vi "Master suppression revised cutoff temp.vi"() -> ()   [LabVIEW 2017]
uses:
  <vilib>/Instr/_visa.llb/VISA Configure Serial Port (Instr).vi
panel:
  in  "Ready for Testing":bool
  in  "Suppression Manual":bool
  out "Suppression Mode":bool
  out "Mode":string
  in  "Suppression Voltage":dbl
  out "Waveform Chart 2":cluster{"U":dbl}(graph)
  out "Total saving Time":dbl
  out "Waveform Chart":cluster{dbl, dbl, dbl}(graph)
  in  "Plotting Rate (ms)":u32=10 min=10 max=100 step=10
  in  "Start/Stop":bool
  out "Boolean":bool
  in  "Sampling Rate(ms)":u32=200 min=200 max=5000
  in  "Baud Rate (9600)":u32=9600
  out "Read Buffer":string
  in  "VISA resource name":refnum<visa-resource-name>
  # "DATA LOGGER with Arduino Mega"
  # "- Select VISA resource name\n- Select Baud Rate\n- Click Arrow Symbol for Start\n- Select Sampling Rate for logger\n- Click START and set name for logger \n- Click STOP to stop SAVE\n- Click Ready for Testing to start\n**Click Suppression Manual for sending \"2\" to Arduino manually"
  # "Sec"
  # "NON COMMERCIAL FOR USE"
  # "Wait for buiding .EXE"
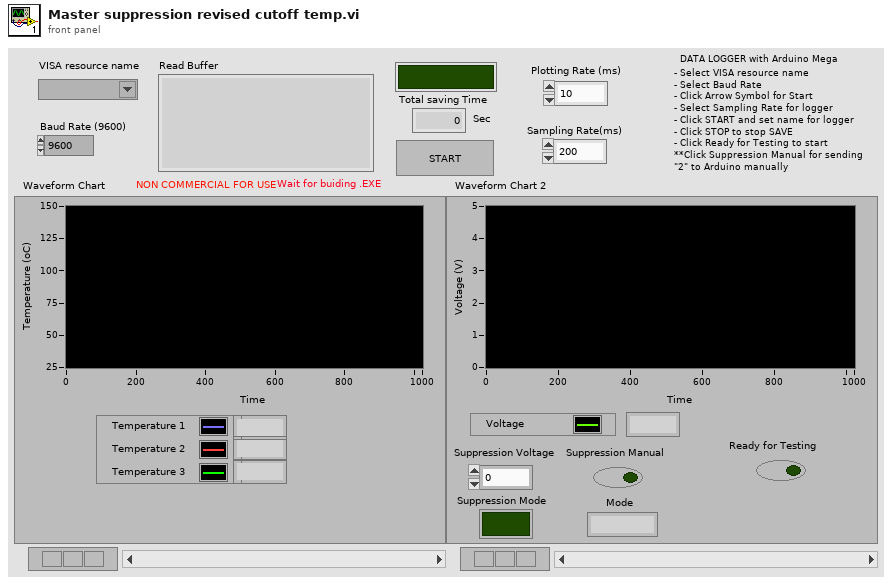
[diagram p1: front panel]
types:
  T1 = enum16{"open", "replace", "create", "open or create", "replace or create", "replace or create with confirmation"}
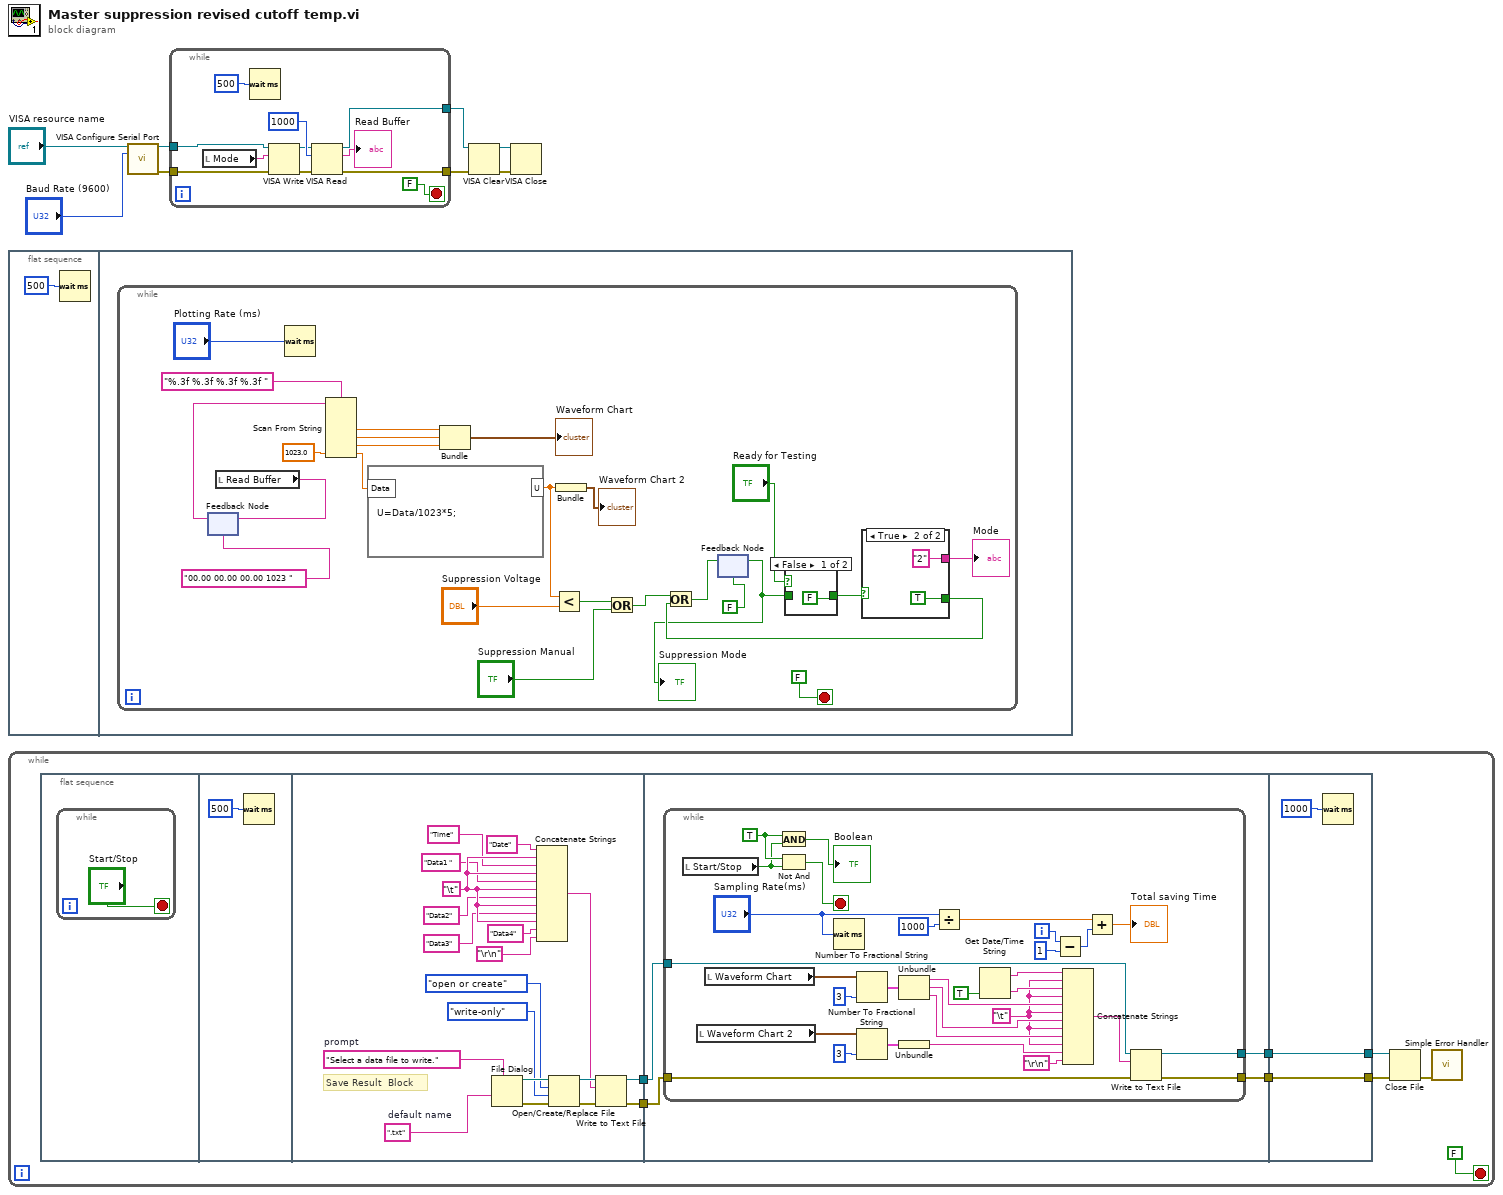
[diagram p0: block diagram]
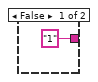
[diagram p3: hidden frame]
diagram:
  n1 = flat-sequence {
    frame #0 {
      n2 = Wait (ms)(milliseconds to wait=u32 500) -> ()  [unwired: 1 out]
    }
    frame #1 {
      n3 = while {
        stop <- FALSE ("OK Button") stop-if-true
        n4 = feedback #1("00.00 00.00 00.00 1023 " ("format string")) -> (w18:string)
        n5 = local read "Read Buffer"() -> (w19:string)
        n6 = feedback-in #1(w19) -> ()
        n7 = Wait (ms)(milliseconds to wait="Plotting Rate (ms)") -> ()  [unwired: 1 out]
        n8 = Scan From String(format string="%.3f %.3f %.3f %.3f ", input string=w18, default 4=1023.0) -> (output 1=w32:dbl, output 2=w31:dbl, output 3=w30:dbl, output 4=w26:dbl)  [unwired: 5 in, 3 out]
        n9 = formula code="U=Data/1023*5;"("Data"=w26) -> ("U"=w25:dbl)
        n10 = Bundle(w32, w31, w30) -> (→"Waveform Chart":cluster{dbl, dbl, dbl})  [unwired: 1 in]
        n11 = Less?(x=w25, y="Suppression Voltage") -> (x < y?=w21:bool)
        n12 = Bundle("U"=w25) -> (→"Waveform Chart 2":cluster{"U":dbl})  [unwired: 1 in]
        n13 = Or(x=w21, y="Suppression Manual") -> (x .or. y?=w16:bool)
        n14 = feedback #2(FALSE) -> (w12:bool)
        "Suppression Mode" <- w12
        n15 = case shown="False" "Ready for Testing" {
          tunnel: w12 -> [_ w36]
          tunnel: [FALSE w36] -> w11
          frame False {
          }
          frame True {
          }
        }
        n16 = case shown="True" w11 {
          tunnel: ["1" "2"] -> w23
          tunnel: [_ TRUE] -> w15
          frame False {
          }
          frame True {
          }
        }
        "Mode" <- w23
        n17 = Or(x=w16, y=w15) -> (x .or. y?=w14:bool)
        n18 = feedback-in #2(w14) -> ()
      }
    }
  }
  n19 = while {
    stop <- FALSE ("OK Button") stop-if-true
    n20 = flat-sequence {
      tunnel: [w52] -> w47
      tunnel: [w51] -> w46
      tunnel: w47 -> [w72]
      tunnel: w46 -> [w71]
      tunnel: [w70] -> w45
      tunnel: [w69] -> w44
      tunnel: [w106] -> w42
      tunnel: w45 -> [w106]
      tunnel: w44 -> [w105]
      tunnel: [w105] -> w41
      frame #0 {
        n21 = while {
          stop <- "Start/Stop" stop-if-true
        }
      }
      frame #1 {
        n22 = Wait (ms)(milliseconds to wait=u32 500) -> ()  [unwired: 1 out]
      }
      frame #2 {
        w60 = ".txt"  # default name
        w61 = "Select a data file to write."  # prompt
        w58 = "\t"
        # "Save Result  Block"
        n23 = File Dialog(7:w61, 9:w60) -> (0:w66:errorcluster, 3:w65:path)  [unwired: 5 in, 2 out]
        n24 = Concatenate Strings("Date", w58, "Time", w58, "Data1 ", w58, "Data2", w58, "Data3", w58, "Data4", "\r\n") -> (w64:string)
        n25 = Open/Create/Replace File(file path (use dialog)=w65, error in=w66, operation (0:open)=T1."open or create", access (0:read/write)=enum16{"read/write", "read-only", "write-only"}."write-only") -> (refnum out=w68:refnum<file>, error out=w67:errorcluster)  [unwired: 2 in, 1 out]
        n26 = Write to Text File(file (use dialog)=w68, text=w64, error in=w67) -> (refnum out=w52:refnum<file>, error out=w51:errorcluster)  [unwired: 1 in, 1 out]
      }
      frame #3 {
        n27 = while {
          tunnel: w72 -> [w103]
          tunnel: w71 -> [w102]
          tunnel: [w101] -> w70
          tunnel: [w100] -> w69
          i -> [w90]
          stop <- w97 stop-if-true
          w78 = "\t"
          w96 = TRUE
          n28 = local read "Start/Stop"() -> (w95:bool)
          n29 = local read "Waveform Chart 2"() -> (w73:cluster{"U":dbl})
          n30 = local read "Waveform Chart"() -> (w85:cluster{dbl, dbl, dbl})
          n31 = And(x=w96, y=w95) -> (x .and. y?=→"Boolean":bool)
          n32 = Not And(1:w95, 2:w96) -> (0:w97:bool)
          n33 = Wait (ms)(milliseconds to wait="Sampling Rate(ms)") -> ()  [unwired: 1 out]
          n34 = Number To Fractional String(number=w85, precision (6)=i16 3) -> (F-format string=w84:cluster{string, string, string})  [unwired: 2 in]
          n35 = Number To Fractional String(number=w73, precision (6)=i16 3) -> (F-format string=w75:cluster{"U":string})  [unwired: 2 in]
          n36 = Unbundle(w84) -> (w81:string, w80:string, w79:string)
          n37 = Unbundle(w75) -> ("U"=w74:string)
          n38 = Divide(x="Sampling Rate(ms)", y=u32 1000) -> (x/y=w92:dbl)
          n39 = Get Date/Time String(want seconds? (F)=TRUE) -> (date string=w83:string, time string=w82:string)  [unwired: 2 in]
          n40 = Subtract(x=w90, y=1) -> (x-y=w89:i32)
          n41 = Concatenate Strings(w83, w78, w82, w78, w81, w78, w80, w78, w79, w78, w74, "\r\n") -> (w87:string)
          n42 = Add(x=w92, y=w89) -> (x+y=→"Total saving Time":dbl)
          n43 = Write to Text File(file (use dialog)=w103, text=w87, error in=w102) -> (refnum out=w101:refnum<file>, error out=w100:errorcluster)  [unwired: 1 in, 1 out]
        }
      }
      frame #4 {
        n44 = Wait (ms)(milliseconds to wait=u32 1000) -> ()  [unwired: 1 out]
      }
    }
    n45 = Close File(refnum=w42, error in=w41) -> (error out=w43:errorcluster)  [unwired: 1 out]
    n46 = call <vilib>:"Simple Error Handler.vi"("error in (no error)"=w43) -> ()  [unwired: 4 in, 5 out]
  }
  n47 = call-poly "VISA Configure Serial Port"("VISA resource name"="VISA resource name", "baud rate (9600)"="Baud Rate (9600)") -> ("VISA resource name out"=w2:refnum<visa-resource-name>, "error out"=w1:errorcluster)  [unwired: 12 in]
  n48 = while {
    tunnel: [w115] -> w3
    tunnel: [w114] -> w4
    tunnel: w2 -> [w111]
    tunnel: w1 -> [w110]
    stop <- FALSE ("Boolean") stop-if-true
    n49 = local read "Mode"() -> (w107:string)
    n50 = Wait (ms)(milliseconds to wait=u32 500 ("Sampling Rate(ms) 2")) -> ()  [unwired: 1 out]
    n51 = VISA Write(VISA resource name=w111, write buffer=w107, error in (no error)=w110) -> (VISA resource name out=w108:refnum<visa-resource-name>, error out=w109:errorcluster)  [unwired: 1 out]
    n52 = VISA Read(VISA resource name=w108, byte count=u32 1000, error in (no error)=w109) -> (VISA resource name out=w115:refnum<visa-resource-name>, read buffer=→"Read Buffer":string, error out=w114:errorcluster)  [unwired: 1 out]
  }
  n53 = VISA Clear(VISA resource name=w3, error in (no error)=w4) -> (VISA resource name out=w7:refnum<visa-resource-name>, error out=w5:errorcluster)
  n54 = VISA Close(VISA resource name=w7, error in (no error)=w5) -> ()  [unwired: 1 out]
